vi "AudioSignalIO.vi"() -> ()   [LabVIEW 2016]
uses:
  <vilib>/Analysis/baseanly.llb/Mean (DBL).vi
  <vilib>/Waveform/WDTOps.llb/WDT Append Waveforms DBL.vi
  <vilib>/Analysis/NI_AALBase.lvlib
panel:
  out "Amplitude Waveform":waveform(dbl)(graph)
  out "Raw Audio\nWaveform":waveform(dbl)(graph)
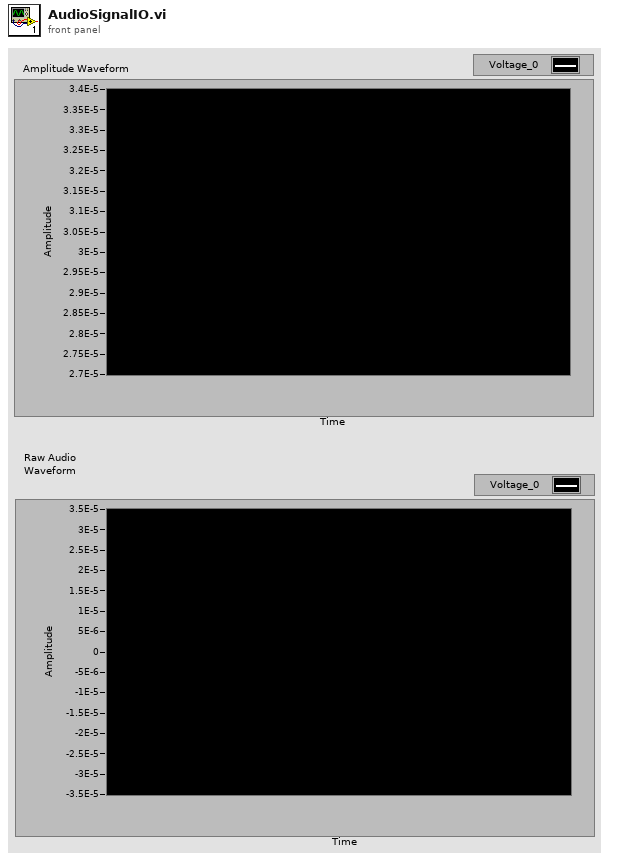
[diagram p1: front panel]
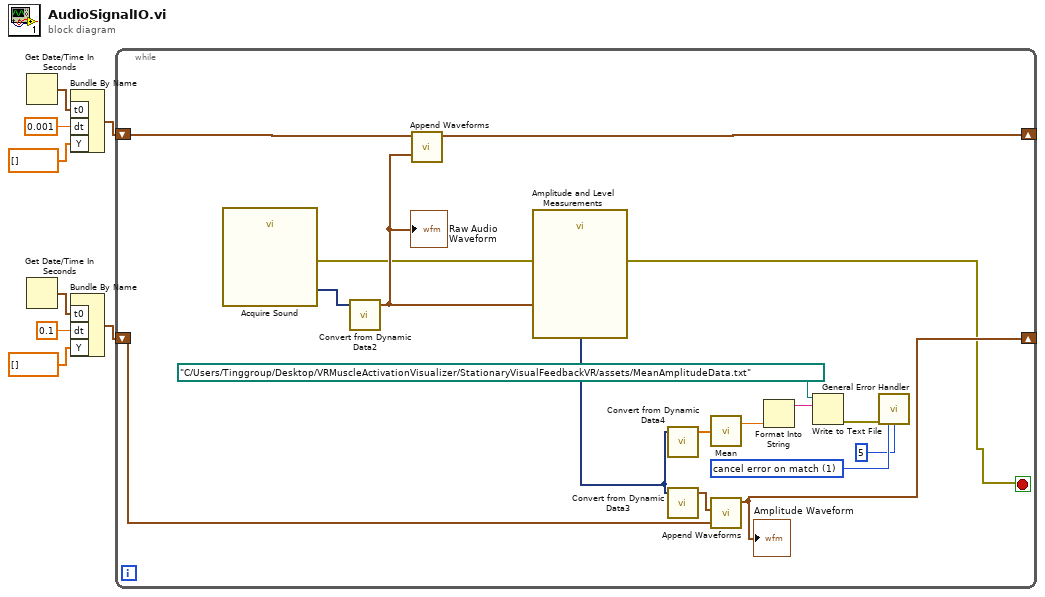
[diagram p0: block diagram]
diagram:
  n1 = Get Date/Time In Seconds() -> (seconds since 1Jan1904=w3:timestamp)
  n2 = Get Date/Time In Seconds() -> (seconds since 1Jan1904=w7:timestamp)
  n3 = Bundle By Name("t0"=w3, "dt"=0.001, "Y"=dbl[] []) -> (w1:waveform(dbl))  [unwired: 1 in]
  n4 = Bundle By Name("t0"=w7, "dt"=0.1, "Y"=dbl[] []) -> (w5:waveform(dbl))  [unwired: 1 in]
  n5 = while {
    shift-right: [w23] -> _
    shift-left: w5 -> [w24]
    shift-right: [w20] -> _
    shift-left: w1 -> [w21]
    stop <- w9 stop-if-true
    w18 = 1 items=["no exception", "cancel error on match", "set error on match"] ("[exception action] (none:0)")
    n6 = call "Acquire Sound"() -> ("Data"=w10:dynamicdata, "error out"=w9:errorcluster)  [unwired: 18 in]
    n7 = call "Convert from Dynamic Data2"("Dynamic Data Type"=w10, "Channel"=w10) -> ("Waveform"=w22:waveform(dbl))  [unwired: 2 in]
    "Raw Audio\nWaveform" <- w22
    n8 = call-poly <vilib>:"Append Waveforms.vi"("waveform B"=w22, "waveform A"=w21) -> ("waveform out"=w20:waveform(dbl))  [unwired: 8 in, 1 out]
    n9 = call "Amplitude and Level Measurements"("Signals"=w22) -> ("Positive Peak"=w13:dynamicdata)  [unwired: 13 in, 1 out]
    n10 = call "Convert from Dynamic Data4"("Dynamic Data Type"=w13) -> ("Array"=w12:dbl[])  [unwired: 3 in]
    n11 = call "Convert from Dynamic Data3"("Dynamic Data Type"=w13) -> ("Waveform"=w14:waveform(dbl))  [unwired: 3 in]
    n12 = call-poly <vilib>:"Mean.vi"("X"=w12) -> ("mean"=w11:dbl)  [unwired: 1 out]
    n13 = call-poly <vilib>:"Append Waveforms.vi"("waveform B"=w14, "waveform A"=w24) -> ("waveform out"=w23:waveform(dbl))  [unwired: 8 in, 1 out]
    "Amplitude Waveform" <- w23
    n14 = Format Into String(w11) -> (resulting string=w16:string)  [unwired: 3 in, 1 out]
    n15 = Write to Text File(file (use dialog)=path "C:/Users/Tinggroup/Desktop/VRMuscleActivationVisualizer/StationaryVisualFeedbackVR/assets/MeanAmplitudeData.txt", text=w16) -> (error out=w19:errorcluster)  [unwired: 2 in, 2 out]
    n16 = call <vilib>:"General Error Handler.vi"("error in (no error)"=w19, "[exception action] (none:0)"=w18, "[exception code]"=5) -> ()  [unwired: 8 in, 5 out]
  }
